vi "SampleRelativeMove.vi"() -> ()   [LabVIEW 2020]
panel:
  out "Steps Per Sec":i32
  out "Steps Per Sec 2":i32
  in  "Relative Steps":i32
  in  "Motor Number":i32=1
  in  "stop":bool
  out "Position Status":i32
  out "error out":errorcluster
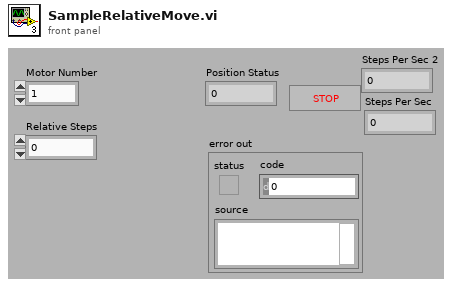
[diagram p1: front panel]
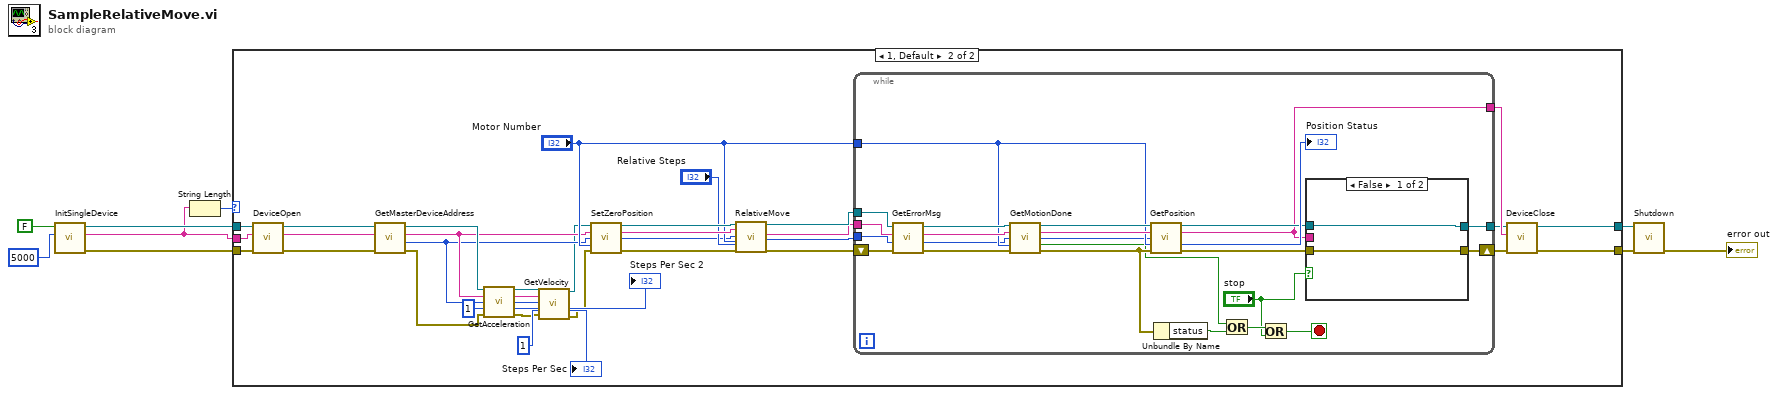
[diagram p0: block diagram]
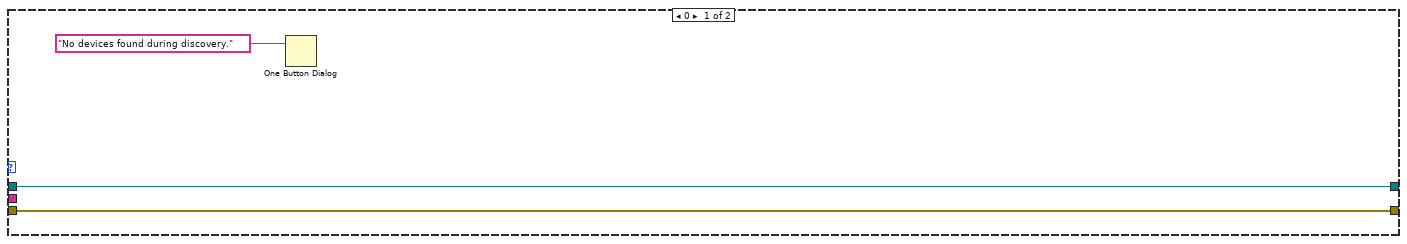
[diagram p2: hidden frame]
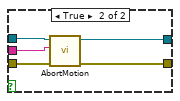
[diagram p3: hidden frame]
diagram:
  n1 = call "InitSingleDevice.vi"("msecDelayForDiscovery"=5000, "logging"=FALSE) -> ("error out"=w1:errorcluster, "DeviceKey Out"=w2:string, "CmdLib Out"=w4:refnum<k24>)  [unwired: 3 in]
  n2 = String Length(string=w2) -> (length=w3:i32)
  n3 = case shown="1, Default" w3 {
    tunnel: [w11 w27] -> w6
    tunnel: [w10 w29] -> w5
    tunnel: w4 -> [w11 w33]
    tunnel: w2 -> [_ w35]
    tunnel: w1 -> [w10 w37]
    frame 0 {
      n4 = One Button Dialog(message="No devices found during discovery.") -> ()  [unwired: 1 in, 1 out]
    }
    frame 1, Default {
      n5 = call "DeviceOpen.vi"("error in (no error)"=w37, "DeviceKey In"=w35, "CmdLib In"=w33) -> ("error out"=w36:errorcluster, "DeviceKey Out"=w34:string, "CmdLib Out"=w32:refnum<k24>)  [unwired: 2 in]
      n6 = call "GetMasterDeviceAddress.vi"("error in (no error)"=w36, "DeviceKey In"=w34, "CmdLib In"=w32) -> ("error out"=w14:errorcluster, "Device Address"=w24:i32, "DeviceKey Out"=w25:string, "CmdLib Out"=w26:refnum<k24>)  [unwired: 1 in]
      n7 = call "GetAcceleration.vi"("CmdLib In"=w26, "DeviceKey In"=w25, "Device Address In"=w24, "Motor"=1, "error in (no error)"=w14) -> ("CmdLib Out"=w22:refnum<k24>, "DeviceKey Out"=w21:string, "Device Address Out"=w20:i32, "Steps Per Sec 2"=→"Steps Per Sec 2":i32, "error out"=w18:errorcluster)  [unwired: 6 in]
      n8 = call "GetVelocity.vi"("CmdLib In"=w22, "DeviceKey In"=w21, "Device Address In"=w20, "Motor"=1, "error in (no error)"=w18) -> ("CmdLib Out"=w15:refnum<k24>, "Steps Per Sec"=→"Steps Per Sec":i32, "error out"=w13:errorcluster)  [unwired: 6 in, 2 out]
      n9 = call "SetZeroPosition.vi"("CmdLib In"=w15, "DeviceKey In"=w25, "Device Address In"=w24, "Motor"="Motor Number", "error in (no error)"=w13) -> ("CmdLib Out"=w44:refnum<k24>, "DeviceKey Out"=w43:string, "Device Address Out"=w39:i32, "error out"=w42:errorcluster)  [unwired: 7 in]
      n10 = call "RelativeMove.vi"("CmdLib In"=w44, "DeviceKey In"=w43, "Device Address In"=w39, "Motor"="Motor Number", "Relative Steps"="Relative Steps", "error in (no error)"=w42) -> ("CmdLib Out"=w47:refnum<k24>, "DeviceKey Out"=w46:string, "Device Address Out"=w38:i32, "error out"=w45:errorcluster)  [unwired: 10 in]
      n11 = while {
        tunnel: "Motor Number" -> [w67]
        tunnel: w47 -> [w66]
        tunnel: w46 -> [w65]
        tunnel: [w52] -> w28
        tunnel: w38 -> [w51]
        shift-right: [w54] -> w30
        shift-left: w45 -> [w64]
        tunnel: [w48] -> w31
        stop <- w57 stop-if-true
        n12 = call "GetErrorMsg.vi"("error in (no error)"=w64, "Device Address In"=w51, "DeviceKey In"=w65, "CmdLib In"=w66) -> ("error out"=w63:errorcluster, "Device Address Out"=w50:i32, "DeviceKey Out"=w69:string, "CmdLib Out"=w68:refnum<k24>)
        n13 = call "GetMotionDone.vi"("CmdLib In"=w68, "DeviceKey In"=w69, "Device Address In"=w50, "Motor"=w67, "error in (no error)"=w63) -> ("CmdLib Out"=w70:refnum<k24>, "DeviceKey Out"=w71:string, "Device Address Out"=w49:i32, "Is Motion Done"=w60:bool, "error out"=w61:errorcluster)  [unwired: 6 in]
        n14 = call "GetPosition.vi"("CmdLib In"=w70, "DeviceKey In"=w71, "Device Address In"=w49, "Motor"=w67, "error in (no error)"=w61) -> ("CmdLib Out"=w53:refnum<k24>, "DeviceKey Out"=w48:string, "Position"=→"Position Status":i32, "error out"=w55:errorcluster)  [unwired: 6 in, 1 out]
        n15 = Unbundle By Name(w61) -> ("status"=w62:bool)
        n16 = Or(x=w60, y=w62) -> (x .or. y?=w58:bool)
        n17 = Or(x=w58, y="stop") -> (x .or. y?=w57:bool)
        n18 = case shown="False" "stop" {
          tunnel: w55 -> [w72 w78]
          tunnel: [w72 w77] -> w54
          tunnel: w53 -> [w73 w76]
          tunnel: [w73 w75] -> w52
          tunnel: w48 -> [_ w74]
          frame False {
          }
          frame True {
            n19 = call "AbortMotion.vi"("error in (no error)"=w78, "DeviceKey In"=w74, "CmdLib In"=w76) -> ("error out"=w77:errorcluster, "CmdLib Out"=w75:refnum<k24>)  [unwired: 1 in, 2 out]
          }
        }
      }
      n20 = call "DeviceClose.vi"("error in (no error)"=w30, "DeviceKey In"=w31, "CmdLib In"=w28) -> ("error out"=w29:errorcluster, "CmdLib Out"=w27:refnum<k24>)  [unwired: 2 in, 1 out]
    }
  }
  n21 = call "Shutdown.vi"("error in (no error)"=w5, "CmdLib In"=w6) -> ("error out"=→"error out":errorcluster)  [unwired: 4 in, 1 out]
